vi "set subpage.vi"(0 "VISA in":refnum<visa-resource-name>, 1 "Location Cluster in":T1, 2 "set subpage":i32, 5 "error in":errorcluster) -> (14 "VISA out":refnum<visa-resource-name>, 15 "Location Cluster out":T1, 19 "error out":errorcluster)   [LabVIEW 2018]
uses:
  location cluster.ctl
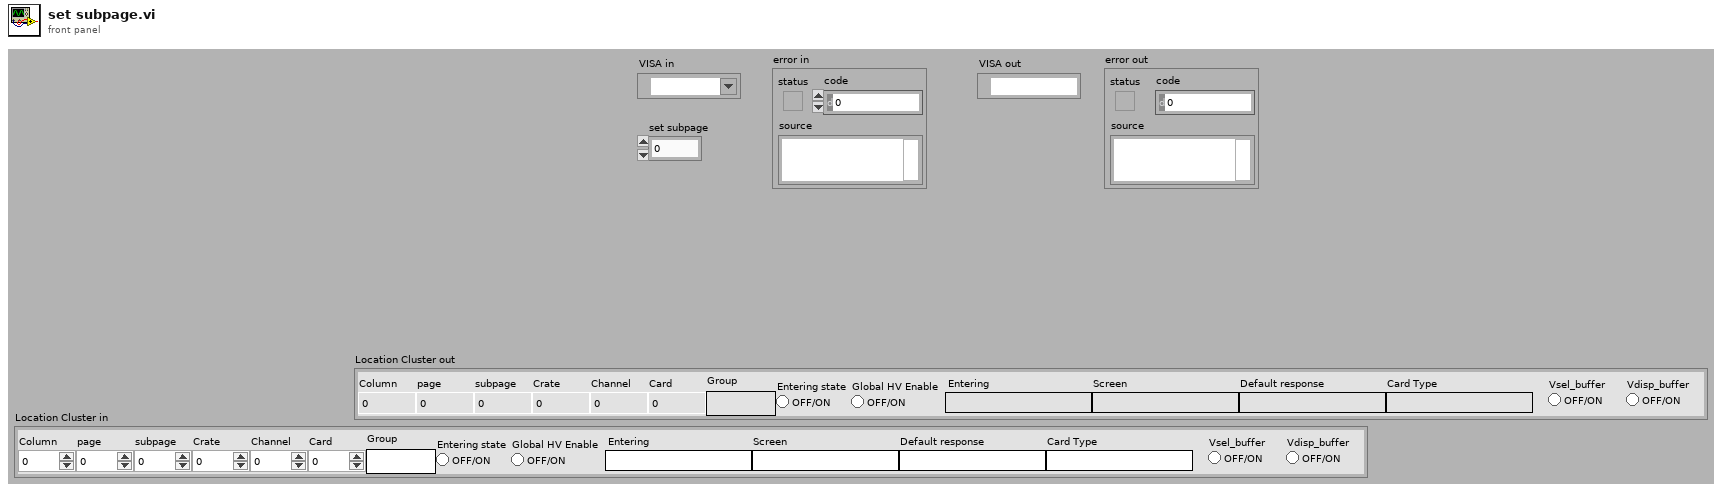
[diagram p1: front panel]
types:
  T1 = typedef "location cluster.ctl" = cluster{"Column":i32, "Card Type":string, "Channel":i32, "Card":i32, "Default response":string, "Entering":string, "Entering state":bool, "subpage":i32, "page":i32, "Crate":i32, "Screen":string, "Group":string, "Global HV Enable":bool, "Vsel_buffer":bool, "Vdisp_buffer":bool}
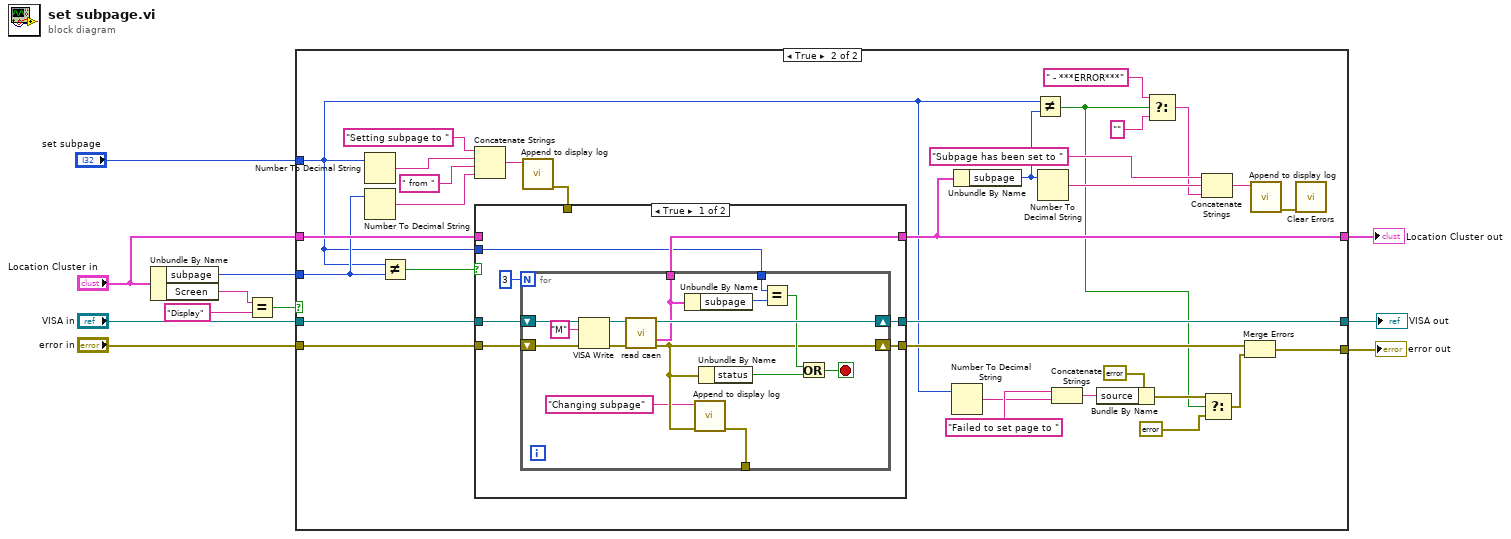
[diagram p0: block diagram]
diagram:
  n1 = Unbundle By Name("Location Cluster in") -> ("subpage"=w5:i32, "Screen"=w6:string)
  n2 = Equal?(x=w6, y="Display" ("x")) -> (x = y?=w1:bool)
  n3 = case shown="True" w1 {
    tunnel: [w12 w46] -> w11
    tunnel: "Location Cluster in" -> [w14 w45]
    tunnel: "error in" -> [w13 w44]
    tunnel: "VISA in" -> [w12 w43]
    tunnel: w5 -> [_ w36]
    tunnel: [w14 w32] -> w4
    tunnel: [w13 w18] -> w3
    tunnel: "set subpage" -> [_ w16]
    frame False {
    }
    frame True {
      n4 = Number To Decimal String(number=w16) -> (decimal integer string=w42:string)  [unwired: 1 in]
      n5 = Number To Decimal String(number=w36) -> (decimal integer string=w41:string)  [unwired: 1 in]
      n6 = Not Equal?(x=w16, y=w36) -> (x != y?=w15:bool)
      n7 = Concatenate Strings("Setting subpage to " ("string"), w42, " from " ("string"), w41) -> (w40:string)
      n8 = call "Append to display log.vi"("string"=w40) -> ("error out"=w39:errorcluster)  [unwired: 10 in]
      n9 = case shown="True" w15 {
        tunnel: w43 -> [w53 w71]
        tunnel: w44 -> [w52 w70]
        tunnel: [w51 w71] -> w46
        tunnel: [w50 w70] -> w19
        tunnel: w45 -> [_ w69]
        tunnel: [w49 w69] -> w32
        tunnel: w39 -> [_ _]
        tunnel: w16 -> [w47 _]
        frame True {
          n10 = for {
            N: 3 -> [_]
            tunnel: [w60] -> w49
            shift-right: [w63] -> w51
            shift-left: w53 -> [w68]
            shift-right: [w56] -> w50
            shift-left: w52 -> [w67]
            tunnel: w47 -> [w58]
            tunnel: [w54] -> _
            stop <- w61 stop-if-true
            n11 = VISA Write(VISA resource name=w68, write buffer="M" ("keys"), error in (no error)=w67) -> (VISA resource name out=w65:refnum<visa-resource-name>, error out=w64:errorcluster)  [unwired: 1 out]
            n12 = call "read caen.vi"("VISA in"=w65, "error in"=w64) -> ("VISA out"=w63:refnum<visa-resource-name>, "Location Cluster"=w60:T1, "error out"=w56:errorcluster)  [unwired: 8 in, 3 out]
            n13 = Unbundle By Name(w60) -> ("subpage"=w59:i32)
            n14 = call "Append to display log.vi"("error in"=w56, "string"="Changing subpage") -> ("error out"=w54:errorcluster)  [unwired: 9 in]
            n15 = Unbundle By Name(w56) -> ("status"=w62:bool)
            n16 = Equal?(x=w58, y=w59) -> (x = y?=w57:bool)
            n17 = Or(x=w57, y=w62) -> (x .or. y?=w61:bool)
          }
        }
        frame False {
        }
      }
      n18 = Number To Decimal String(number=w16) -> (decimal integer string=w20:string)  [unwired: 1 in]
      n19 = Unbundle By Name(w32) -> ("subpage"=w28:i32)
      n20 = Not Equal?(x=w16, y=w28) -> (x != y?=w17:bool)
      n21 = Number To Decimal String(number=w28) -> (decimal integer string=w33:string)  [unwired: 1 in]
      n22 = Concatenate Strings("Failed to set page to " ("string"), w20) -> (w22:string)
      n23 = Bundle By Name(cluster=errorcluster {"status"=TRUE, "code"=0, "source"=""} ("error in"), "source"=w22) -> (w23:errorcluster)
      n24 = Select(t=" - ***ERROR***" ("string"), s=w17, f="" ("string")) -> (s? t:f=w27:string)
      n25 = Concatenate Strings("Subpage has been set to " ("string"), w33, w27) -> (w34:string)
      n26 = Select(t=w23, s=w17, f=errorcluster {"status"=FALSE, "code"=0, "source"=""} ("error in")) -> (s? t:f=w26:errorcluster)
      n27 = Merge Errors(w19, w26) -> (w18:errorcluster)
      n28 = call "Append to display log.vi"("string"=w34) -> ("error out"=w31:errorcluster)  [unwired: 10 in]
      n29 = call <vilib>:"Clear Errors.vi"("error in (no error)"=w31) -> ()  [unwired: 5 in, 2 out]
    }
  }
  "Location Cluster out" <- w4
  "error out" <- w3
  "VISA out" <- w11
